vi "Initialize.vi"(0 "File in":refnum<class "File.lvclass">, 1 "Filter in":refnum<class "Filter.lvclass">, 5 "Level in":refnum<class "Level.lvclass">, 7 "Fs (Hz)":dbl, 9 "Npts":i32, 11 "error in (no error)":errorcluster, 13 "Channel Name":string) -> (3 "Filter out":refnum<class "Filter.lvclass">, 4 "File out":refnum<class "File.lvclass">, 6 "Level out":refnum<class "Level.lvclass">, 15 "error out":errorcluster)   [LabVIEW 2020, in "File.lvclass"]
uses:
  File.lvclass
  Level/Level.lvclass
  Filter/Filter.lvclass
  File.lvclass/File.ctl
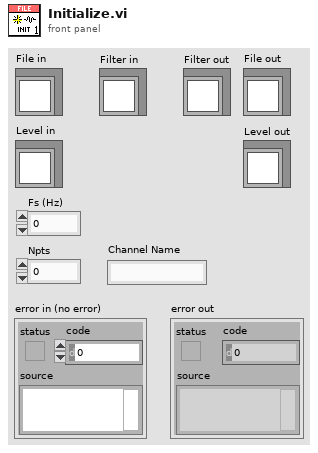
[diagram p1: front panel]
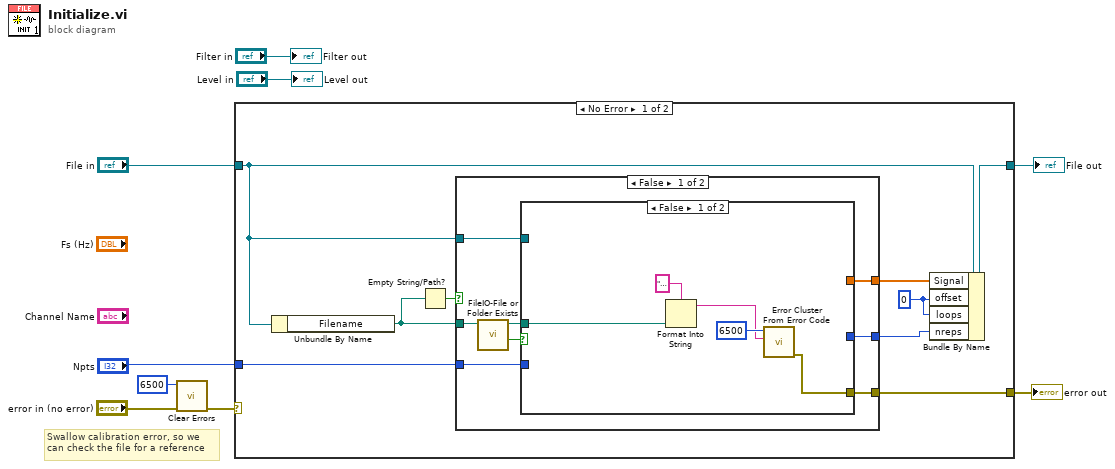
[diagram p0: block diagram]
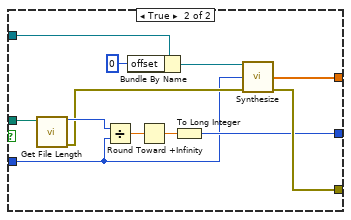
[diagram p2: hidden frame]
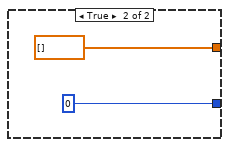
[diagram p3: hidden frame]
diagram:
  # "Swallow calibration error, so we \ncan check the file for a reference"
  n1 = call <vilib>:"Clear Errors.vi"("error in (no error)"="error in (no error)", "specific error code to clear (0: all)"=6500) -> ("error out"=w2:errorcluster)  [unwired: 4 in, 1 out]
  n2 = case shown="No Error" w2 {
    selector: w2 -> [_ w47]
    tunnel: [w11 w47] -> w9
    tunnel: [w12 w46] -> w8
    tunnel: "File in" -> [w13 w46]
    tunnel: "Npts" -> [w10 _]
    frame No Error {
      w18 = 0 ("offset")
      n3 = Unbundle By Name(w13) -> ("Filename"=w16:path)
      n4 = Empty String/Path?(string/path=w16) -> (empty?=w15:bool)
      n5 = case shown="False" w15 {
        tunnel: w16 -> [w21 _]
        tunnel: [w24 _] -> w11
        tunnel: w10 -> [w22 _]
        tunnel: [w25 dbl[] [] ("Y")] -> w14
        tunnel: [w23 0] -> w17
        tunnel: w13 -> [w26 _]
        frame False {
          n6 = call "FileIO-File or Folder Exists.vi"("path"=w21) -> ("Exists?"=w19:bool, "dup path"=w20:path)  [unwired: 7 in, 2 out]
          n7 = case shown="False" w19 {
            tunnel: w26 -> [_ w40]
            tunnel: [_ w38] -> w25
            tunnel: [w27 w36] -> w24
            tunnel: [_ w35] -> w23
            tunnel: w22 -> [_ w34]
            tunnel: w20 -> [w28 w32]
            frame False {
              n8 = Format Into String(format string="File not found: %s" ("error message (\"\")"), w28) -> (resulting string=w29:string)  [unwired: 2 in, 1 out]
              n9 = call <vilib>:"Error Cluster From Error Code.vi"("error message (\"\")"=w29, "error code (0)"=6500) -> ("error out"=w27:errorcluster)  [unwired: 7 in]
            }
            frame True {
              n10 = call "Get File Length.vi"("Filename"=w32) -> ("total number of samples/ch"=w43:u32, "error out"=w37:errorcluster)  [unwired: 13 in]
              n11 = Divide(x=w43, y=w34) -> (x/y=w42:dbl)
              n12 = Bundle By Name(cluster=w40, "offset"=0) -> (w33:refnum<class "File.lvclass">)
              n13 = Round Toward +Infinity(x=w42) -> (ceil(x): smallest int >= x=w41:dbl)
              n14 = To Long Integer(number=w41) -> (32bit integer=w35:i32)
              n15 = call-dynamic "Synthesize.vi"("File in"=w33, "Npts"=w34, "error in (no error)"=w37) -> ("Array"=w38:dbl[], "error out"=w36:errorcluster)  [unwired: 10 in, 1 out]
            }
          }
        }
        frame True {
        }
      }
      n16 = Bundle By Name(cluster=w13, "Signal"=w14, "offset"=w18, "loops"=w18, "nreps"=w17) -> (w12:refnum<class "File.lvclass">)
    }
    frame Error {
    }
  }
  "error out" <- w9
  "File out" <- w8
  "Level out" <- "Level in"
  "Filter out" <- "Filter in"
